vi "Get Answers Data.vi"(6 "error in (no error)":errorcluster, 8 "data":u32[](array[numeric]), 9 "length":u32) -> (0 "error out":errorcluster, 2 "data out":u32[](array[numeric]), 3 "function return":bool)   [LabVIEW 2015, in "XGL_DPP.lvlib"]
doc: "EXTERN DECLSPEC bool CALL_CONV GetAnswersData(unsigned int length, unsigned int* data);"
uses:
  XGL_DPP.lvlib
  XGL_DPP.dll
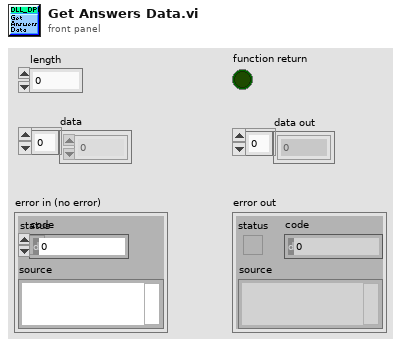
[diagram p1: front panel]
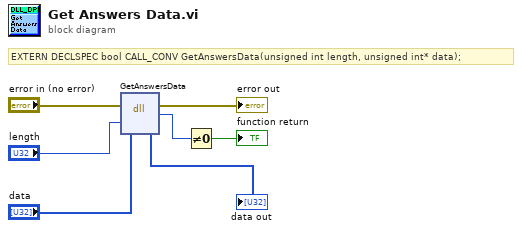
[diagram p0: block diagram]
diagram:
  # "EXTERN DECLSPEC bool CALL_CONV GetAnswersData(unsigned int length, unsigned int* data);"
  n1 = dll-call lib="D:/Users/XRF/Desktop/Dante_acquire4/libs/Dante/XGL_DPP.*" fn="GetAnswersData"(error in="error in (no error)", "length"="length", "data"="data") -> (error out=→"error out":errorcluster, "return type"=w6:u8, "data"=→"data out":u32[])  [unwired: 3 in, 1 out]
  n2 = Not Equal To 0?(x=w6) -> (x != 0?=→"function return":bool)
